vi "meth.StopOutputLoop.vi"(0 "class.GLue in":refnum<class "class.GLue.lvclass">, 2 "ReaderContext in":T1, 11 "error in":errorcluster) -> (4 "class.GLue out":refnum<class "class.GLue.lvclass">, 15 "error out":errorcluster)   [LabVIEW 2014, in "GLue.lvlib" / "class.GLue.lvclass"]
uses:
  class.GLue.lvclass
  class.GLue.lvclass/class.GLue.ctl
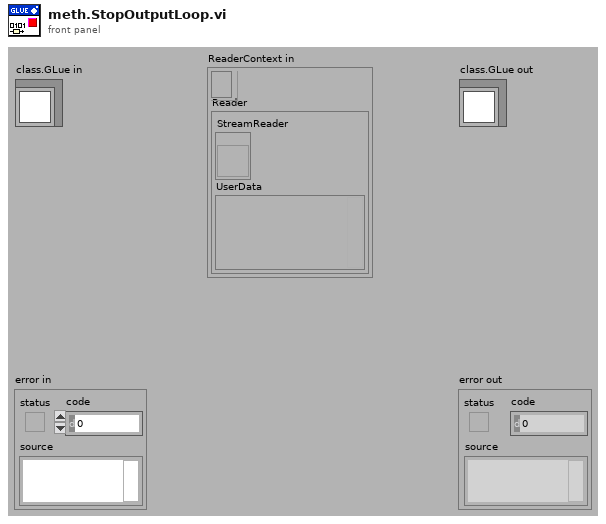
[diagram p1: front panel]
types:
  T1 = cluster{"EventRef":refnum<event-registration>, "Reader":cluster{"StreamReader":refnum<vi>, "UserData":variant}}
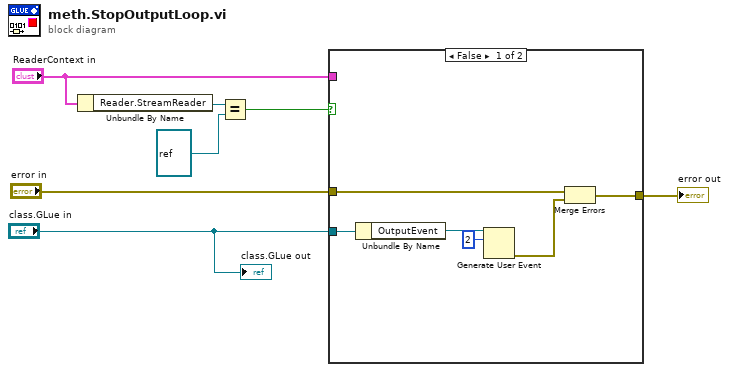
[diagram p0: block diagram]
diagram:
  n1 = Unbundle By Name("ReaderContext in") -> ("Reader.StreamReader"=w2:refnum<vi>)
  n2 = Equal?(x=w2, y=refnum<vi> refnum ("Reader.StreamReader")) -> (x = y?=w1:bool)
  n3 = case shown="False" w1 {
    tunnel: "class.GLue in" -> [w13 _]
    tunnel: "error in" -> [w9 w14]
    tunnel: [w8 w14] -> w6
    tunnel: "ReaderContext in" -> [_ _]
    frame False {
      n4 = Unbundle By Name(w13) -> ("OutputEvent"=w12:refnum<user-event>)
      n5 = Generate User Event(user event=w12, event data cluster=2 ("event data")) -> (error out=w10:errorcluster)  [unwired: 2 in, 1 out]
      n6 = Merge Errors(w9, w10) -> (w8:errorcluster)
    }
    frame True {
    }
  }
  "error out" <- w6
  "class.GLue out" <- "class.GLue in"
